vi "Simple TCP - Client.vi"() -> ()   [LabVIEW 2021]
doc: "Demonstrates how to open a connection to an TCP server, read the data being sent, and display the data on a chart. This VI is designed to stop if the TCP connection is terminated."
uses:
  <vilib>/Analysis/3filter.llb/Butterworth Filter (DBL).vi
  <vilib>/Analysis/NI_AALBase.lvlib
  <vilib>/ptbypt/NI_PtbyPt.lvlib
panel:
  in  "error in (no error)":errorcluster
  in  "Boolean":bool
  out "Waveform Graph 2":dynamicdata(graph)
  out "Waveform Graph 3":dbl[](graph)
  out "Waveform Graph 4":dynamicdata(graph)
  out "Waveform Graph 5":dynamicdata(graph)
  out "Waveform Graph 6":dynamicdata(graph)
  out "Array Size":u32
  out "Waveform Graph 7":dynamicdata(graph)
  out "Waveform Graph 10":dynamicdata(graph)
  out "Array Size 3":u32
  in  "Server Closed":string="The server VI closed the connection."
  out "Waveform Graph":dbl[](graph)
  in  "Stop":bool
  # "Overview: Demonstrates the use of the TCP functions to connect to a TCP server VI and receive data.\nInstructions:\n1. Ensure Simple TCP - Server.vi is already running.\n2. Run the VI.\n3. Click Stop to stop the VI. Note that if you stop the server VI, this VI will stop automatically."
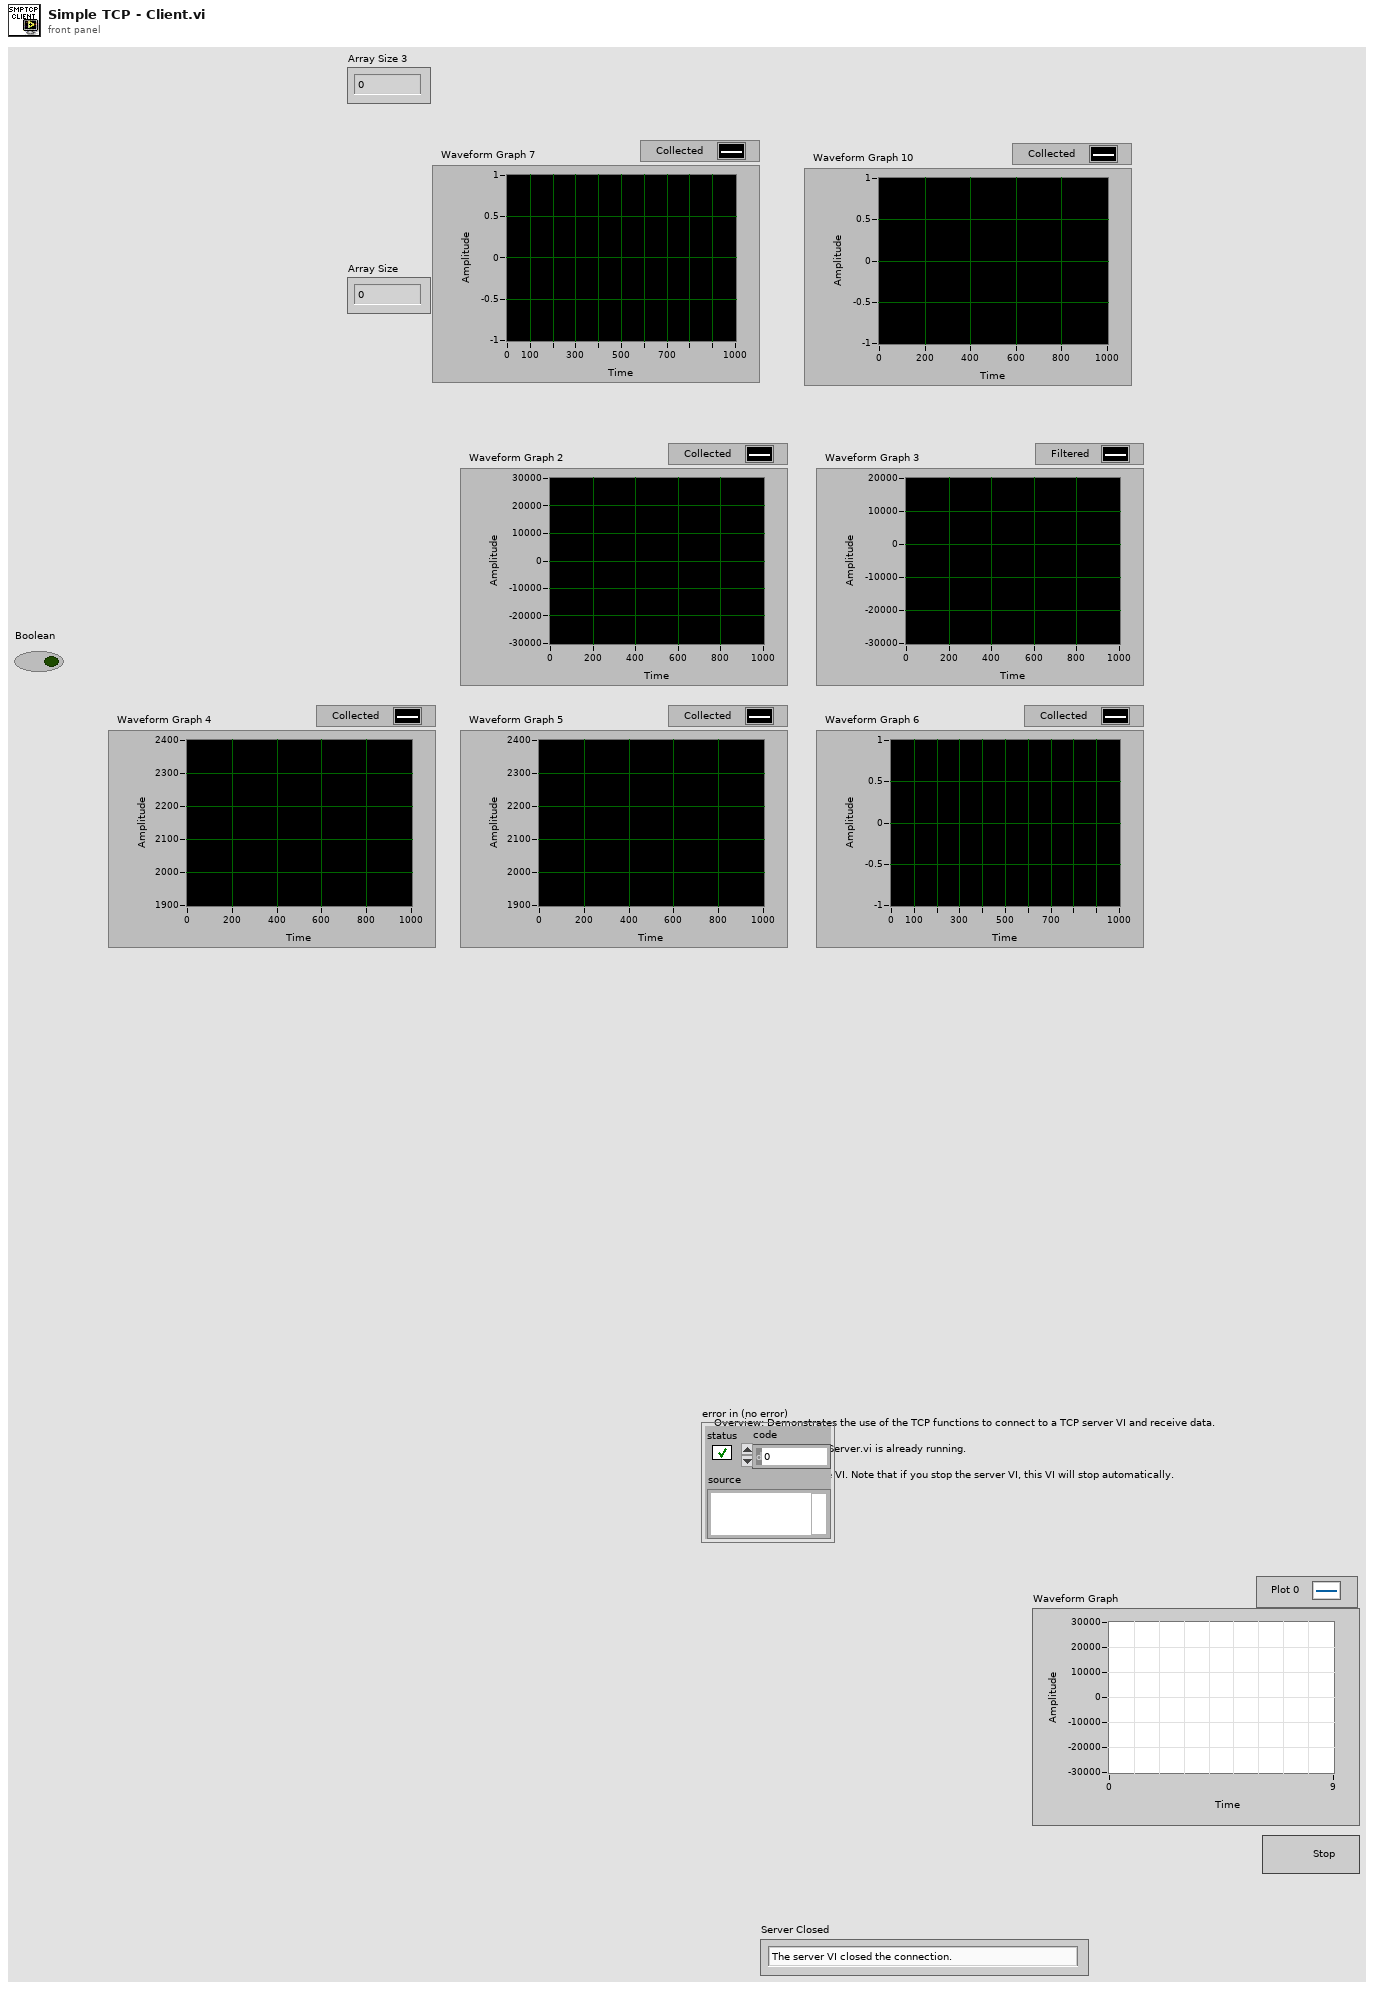
[diagram p1: front panel]
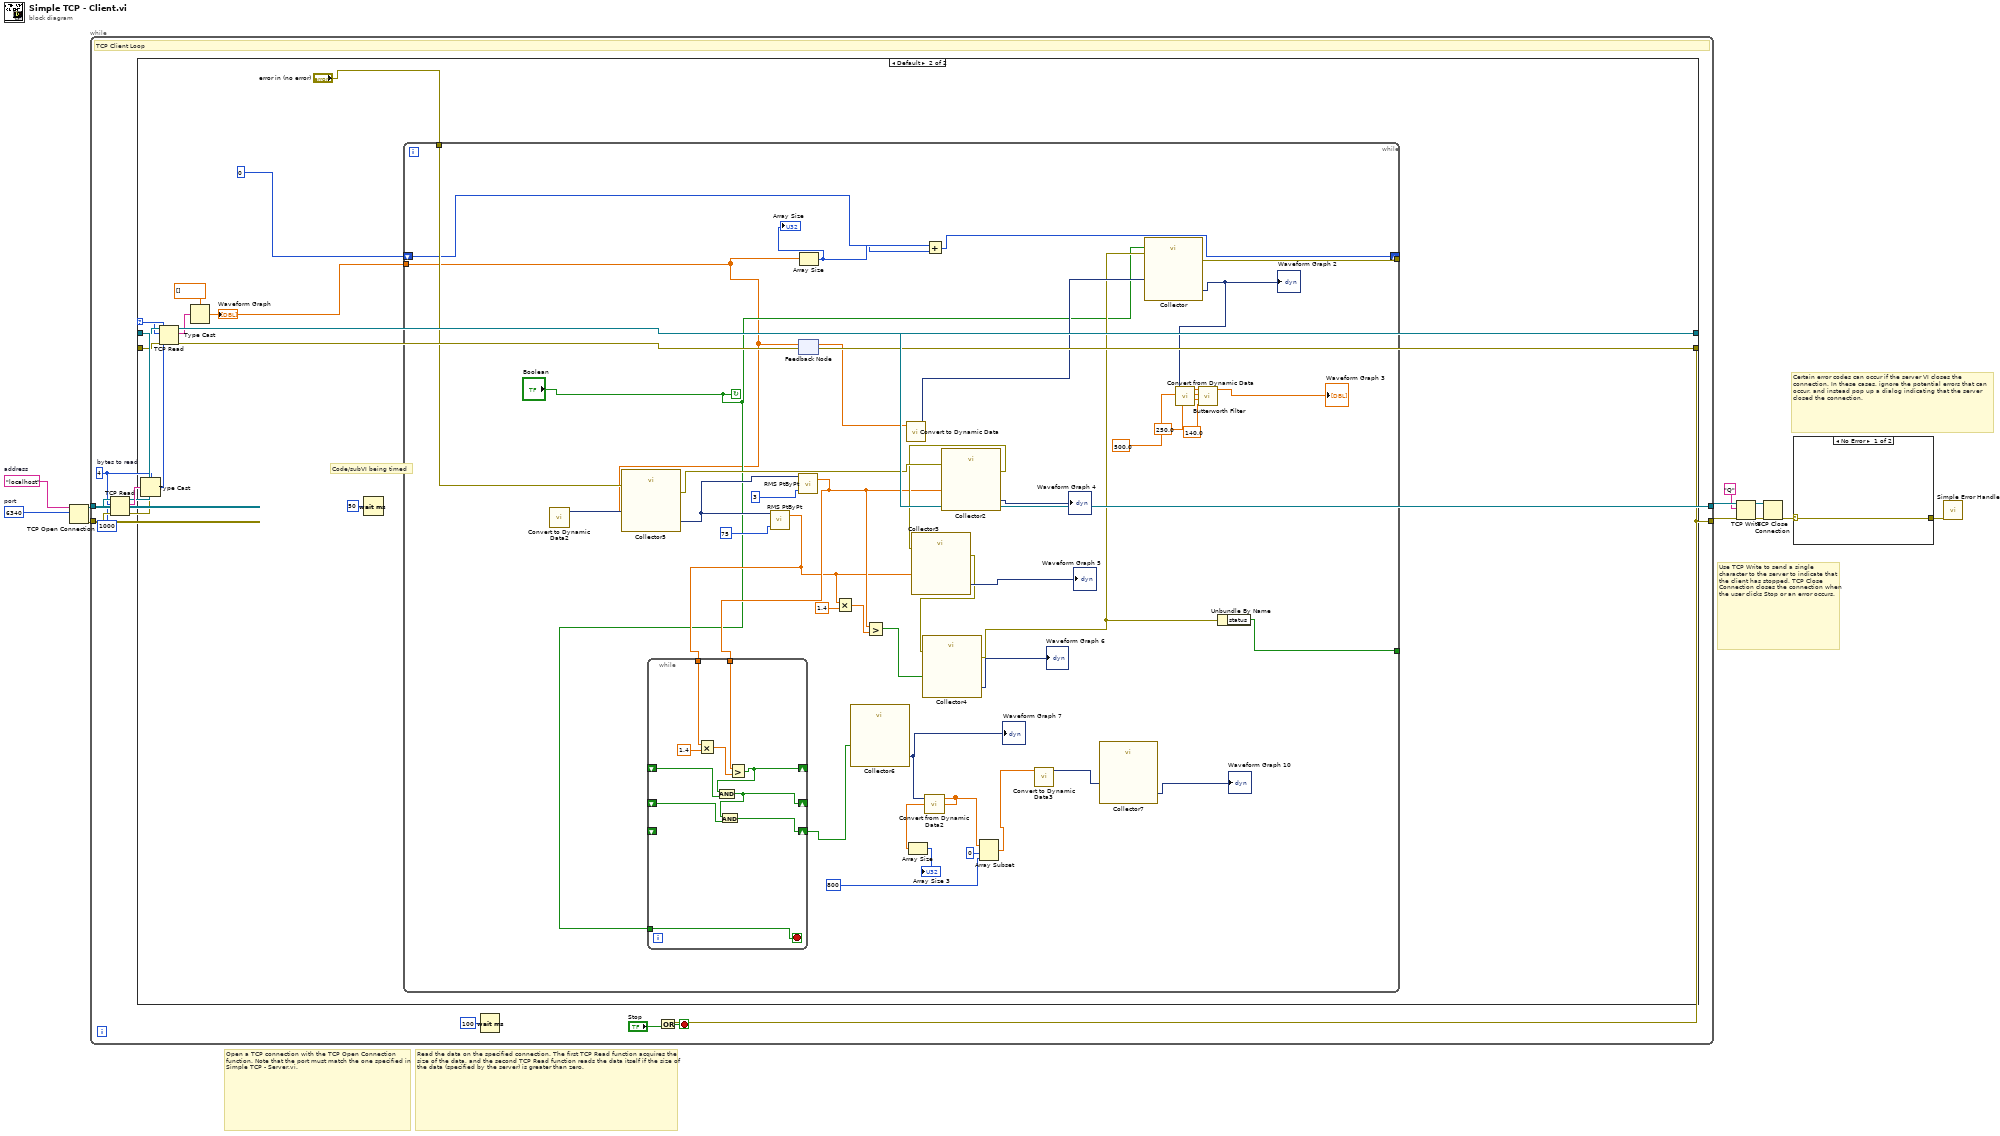
[diagram p0: block diagram]
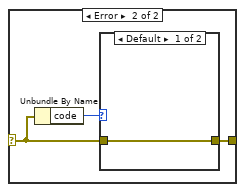
[diagram p2: hidden frame]
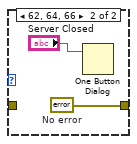
[diagram p3: hidden frame]
diagram:
  w1 = u16 6340  # port
  w2 = "localhost"  # address
  # "Certain error codes can occur if the server VI closes the connection. In these cases, ignore the potential errors that can occur, and instead pop up a dialog indicating that the server closed the connection."
  # "Use TCP Write to send a single character to the server to indicate that the client has stopped. TCP Close Connection closes the connection when the user clicks Stop or an error occurs."
  # "Read the data on the specified connection. The first TCP Read function acquires the size of the data, and the second TCP Read function reads the data itself if the size of the data (specified by the server) is greater than zero."
  # "Open a TCP connection with the TCP Open Connection function. Note that the port must match the one specified in Simple TCP - Server.vi."
  n1 = TCP Open Connection(address=w2, remote port or service name=w1) -> (connection ID=w11:refnum<k5>, error out=w10:errorcluster)  [unwired: 3 in]
  n2 = while {
    tunnel: w10 -> [w20]
    tunnel: w11 -> [w21]
    tunnel: [w15] -> w8
    tunnel: [w14] -> w6
    stop <- w17 stop-if-true
    w19 = 4  # bytes to read
    # "TCP Client Loop"
    n3 = TCP Read(connection ID=w21, bytes to read=w19, error in (no error)=w20, 9:1000 ("timeout ms (25000)")) -> (connection ID out=w23:refnum<k5>, data out=w24:string, error out=w22:errorcluster)  [unwired: 1 in]
    n4 = Type Cast(type=w19, x=w24) -> (*(type *) &x=w13:i32)
    n5 = case shown="Default" w13 {
      selector: w13 -> [_ w31]
      tunnel: w23 -> [w26 w37]
      tunnel: w22 -> [w25 w36]
      tunnel: [w26 w34] -> w15
      tunnel: [w25 w33] -> w14
      frame ..0 {
        # "The server has not written any data"
      }
      frame Default {
        # "Code/subVI being timed"
        n6 = TCP Read(connection ID=w37, bytes to read=w31, error in (no error)=w36) -> (connection ID out=w34:refnum<k5>, data out=w32:string, error out=w33:errorcluster)  [unwired: 2 in]
        n7 = Type Cast(type=dbl[] [] ("chart"), x=w32) -> (*(type *) &x=w27:dbl[])
        "Waveform Graph" <- w27
        n8 = Wait (ms)(milliseconds to wait=u32 50) -> ()  [unwired: 1 out]
        n9 = while {
          tunnel: "error in (no error)" -> [w61]
          tunnel: [w57] -> _
          tunnel: [w55] -> _
          shift-right: [w51] -> _
          shift-left: 0 -> [w52]
          tunnel: w27 -> [w38]
          stop <- "Boolean" continue-if-true
          n10 = call "Convert to Dynamic Data2"("Array"=w38) -> ("Dynamic Data Type"=w63:dynamicdata)  [unwired: 3 in]
          n11 = call "Collector5"("error in (no error)"=w61, "Signals"=w63) -> ("error out"=w60:errorcluster, "Collected Signals"=w62:dynamicdata)  [unwired: 8 in]
          n12 = call <vilib>:"RMS PtByPt.vi"("sample length"=75, "x"=w62) -> ("rms value"=w49:dbl)  [unwired: 2 in, 1 out]
          n13 = call <vilib>:"RMS PtByPt.vi"("sample length"=3, "x"=w62) -> ("rms value"=w50:dbl)  [unwired: 2 in, 1 out]
          n14 = while {
            tunnel: w50 -> [w86]
            tunnel: w49 -> [w85]
            shift-right: [w80] -> _
            shift-left: _ -> [w81]
            shift-right: [w83] -> _
            shift-left: _ -> [w82]
            tunnel: "Boolean" -> [w84]
            shift-right: [w79] -> w46
            shift-left: _ -> [_]
            stop <- w84 stop-if-true
            n15 = Multiply(x=w85, y=1.4) -> (x*y=w87:dbl)
            n16 = Greater?(x=w86, y=w87) -> (0:w83:bool)
            n17 = And(x=w83, y=w82) -> (x .and. y?=w80:bool)
            n18 = And(x=w80, y=w81) -> (x .and. y?=w79:bool)
          }
          n19 = feedback-in #1(w38) -> ()
          n20 = feedback #1() -> (w54:dbl[])  [unwired: 1 in]
          n21 = Array Size(array=w38) -> (size(s)=w53:i32)
          "Array Size" <- w53
          n22 = Multiply(x=w49, y=1.4) -> (x*y=w66:dbl)
          n23 = call "Collector6"("Signals"=w46) -> ("Collected Signals"=w44:dynamicdata)  [unwired: 9 in, 1 out]
          "Waveform Graph 7" <- w44
          n24 = Greater?(x=w50, y=w66) -> (0:w65:bool)
          n25 = call "Convert to Dynamic Data"("Array"=w54) -> ("Dynamic Data Type"=w70:dynamicdata)  [unwired: 3 in]
          n26 = call "Convert from Dynamic Data2"("Dynamic Data Type"=w44) -> ("Array"=w41:dbl[])  [unwired: 3 in]
          n27 = Array Size(array=w41) -> (size(s)=→"Array Size 3":i32)
          n28 = Add(x=w53, y=w52) -> (x+y=w51:i32)
          n29 = call "Collector2"("error in (no error)"=w60, "Signals"=w50) -> ("error out"=w59:errorcluster, "Collected Signals"=→"Waveform Graph 4":dynamicdata)  [unwired: 8 in]
          n30 = call "Collector3"("error in (no error)"=w59, "Signals"=w49) -> ("error out"=w58:errorcluster, "Collected Signals"=→"Waveform Graph 5":dynamicdata)  [unwired: 8 in]
          n31 = call "Collector4"("error in (no error)"=w58, "Signals"=w65) -> ("error out"=w56:errorcluster, "Collected Signals"=→"Waveform Graph 6":dynamicdata)  [unwired: 8 in]
          n32 = Array Subset(array=w41, index=0, length=800 ("index")) -> (w39:dbl[])
          n33 = call "Convert to Dynamic Data3"("Array"=w39) -> ("Dynamic Data Type"=w45:dynamicdata)  [unwired: 3 in]
          n34 = call "Collector7"("Signals"=w45) -> ("Collected Signals"=→"Waveform Graph 10":dynamicdata)  [unwired: 9 in, 1 out]
          n35 = call "Collector"("error in (no error)"=w56, "Enable"="Boolean", "Signals"=w70) -> ("error out"=w57:errorcluster, "Collected Signals"=w73:dynamicdata)  [unwired: 7 in]
          "Waveform Graph 2" <- w73
          n36 = call "Convert from Dynamic Data"("Dynamic Data Type"=w73) -> ("Array"=w75:dbl[])  [unwired: 3 in]
          n37 = call-poly <vilib>:"Butterworth Filter.vi"("low cutoff freq: fl"=140.0, "high cutoff freq: fh"=250.0, "sampling freq: fs"=500.0, "X"=w75) -> ("Filtered X"=→"Waveform Graph 3":dbl[])  [unwired: 4 in, 1 out]
          n38 = Unbundle By Name(w56) -> ("status"=w55:bool)
        }
      }
    }
    n39 = Wait (ms)(milliseconds to wait=u32 100) -> ()  [unwired: 1 out]
    n40 = Or(x=w14, y="Stop") -> (x .or. y?=w17:bool)
  }
  n41 = TCP Write(connection ID=w8, data in="Q", error in (no error)=w6) -> (connection ID out=w9:refnum<k5>, error out=w7:errorcluster)  [unwired: 2 out]
  n42 = TCP Close Connection(connection ID=w9, error in (no error)=w7) -> (error out=w4:errorcluster)  [unwired: 1 in, 1 out]
  n43 = case shown="No Error" w4 {
    selector: w4 -> [w89 w91]
    tunnel: [w89 w90] -> w3
    frame No Error {
    }
    frame Error {
      n44 = Unbundle By Name(w91) -> ("code"=w92:i32)
      n45 = case shown="Default" w92 {
        tunnel: w91 -> [w93 _]
        tunnel: [w93 w95] -> w90
        frame Default {
        }
        frame 62, 64, 66 {
          w95 = errorcluster {"status"=FALSE, "code"=0, "source"=""}  # No error
          n46 = One Button Dialog(message="Server Closed") -> ()  [unwired: 1 in, 1 out]
        }
      }
    }
  }
  n47 = call <vilib>:"Simple Error Handler.vi"("error in (no error)"=w3) -> ()  [unwired: 4 in, 5 out]
